vi "Read Running Actors.vi"(8 "error in (no error)":errorcluster, 11 "cRIO-CO2 in":refnum<class "cRIO-CO2.lvclass">) -> (0 "error out":errorcluster, 2 "Running Actors":refnum<class "CO2 Actor.lvclass">[](array[class]), 3 "cRIO-CO2 out":refnum<class "cRIO-CO2.lvclass">)   [LabVIEW 2015, in "cRIO-Carbondioxide.lvlib" / "cRIO-CO2.lvlib" / "cRIO-CO2.lvclass"]
uses:
  cRIO-CO2.lvclass
  CO2 Actor/CO2 Actor.lvclass
  cRIO-CO2.lvclass/cRIO-CO2.ctl
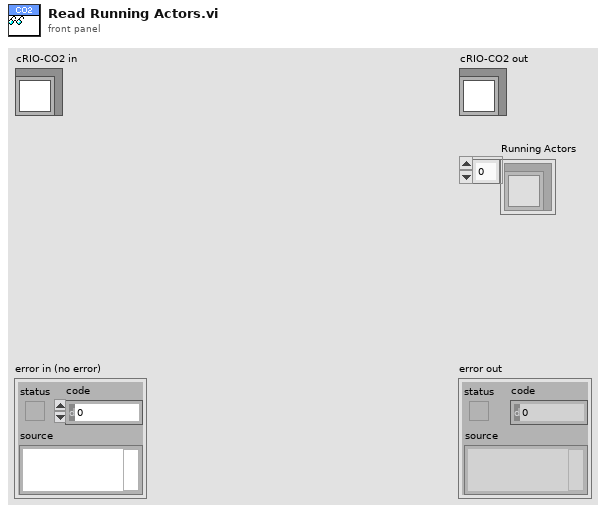
[diagram p1: front panel]
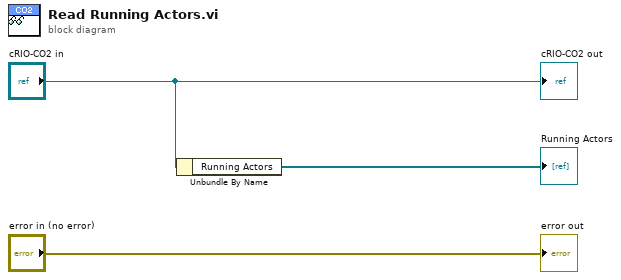
[diagram p0: block diagram]
diagram:
  n1 = Unbundle By Name("cRIO-CO2 in") -> ("Running Actors"=→"Running Actors":refnum<class "CO2 Actor.lvclass">[])
  "error out" <- "error in (no error)"
  "cRIO-CO2 out" <- "cRIO-CO2 in"
